vi "Update Calibration.vi"() -> ()   [LabVIEW 2019]
doc: "This VI implements the framework and scheduler for your robotics program. It should not be necessary to modify the framework. You are expected to add your code to the VIs called from Robot Main - the ones located in the Team Code folder within the project."
uses:
  Robot Global Data.vi
panel:
  in  "Color":string(combo)="Red"
  in  "Set Color":bool
  out "Matched Color Name":string
  out "Match Confidence":dbl
  out "Measured Color":cluster{"R":dbl, "G":dbl, "B":dbl}
  in  "Blue Cal":cluster{"R":dbl, "G":dbl, "B":dbl}={"R"=0.143, "G"=0.427, "B"=0.429} caption="Blue Calibration"
  in  "Green Cal":cluster{"R":dbl, "G":dbl, "B":dbl}={"R"=0.197, "G"=0.561, "B"=0.24} caption="Green Calibration"
  in  "Red Cal":cluster{"R":dbl, "G":dbl, "B":dbl}={"R"=0.561, "G"=0.323, "B"=0.114} caption="Red Calibration"
  in  "Yellow Cal":cluster{"R":dbl, "G":dbl, "B":dbl}={"R"=0.361, "G"=0.524, "B"=0.113} caption="Yellow Calibration"
  out "error out":errorcluster
  out "Proximity":u16(graph)
  out "Color":u32(colorbox)
  in  "Finish":bool
  # "To save calibration:\n\nEdit --> Make Current Values Default"
  # "------>"
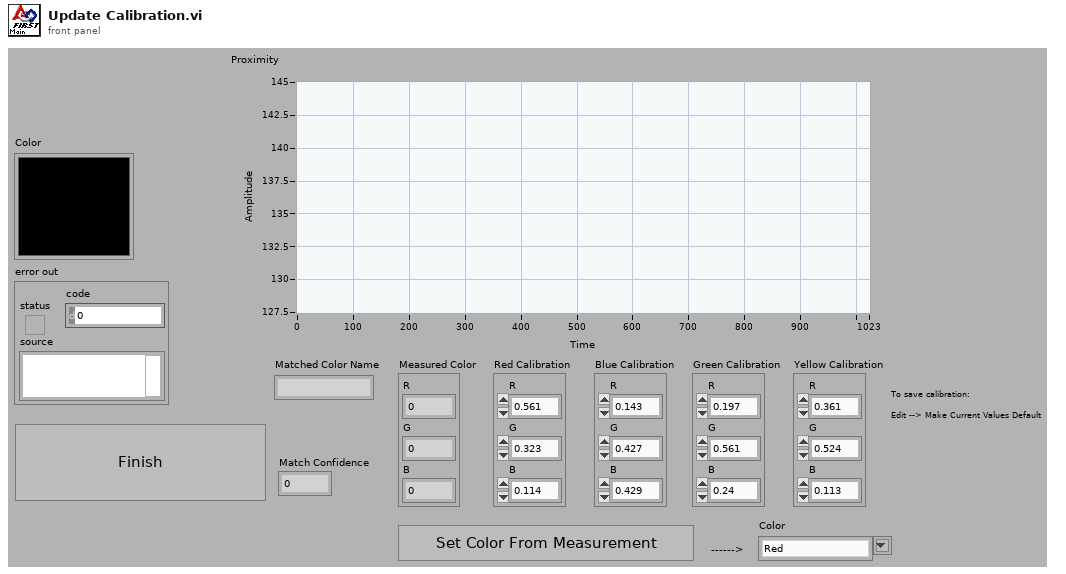
[diagram p1: front panel]
types:
  T1 = typedef "Color Sensor V3 DevRef.ctl" = cluster{"I2CDevRef":T2}
  T2 = typedef "WPI_I2CDevRef.ctl" = cluster{"DevStatus":errorcluster, "Device Address":u8, "Handle":i32, "I2C Bus":T3}
  T3 = typedef "i2c_bus.ctl" = enum16{"I2C On-Board", "I2C MXP", "Invalid"}
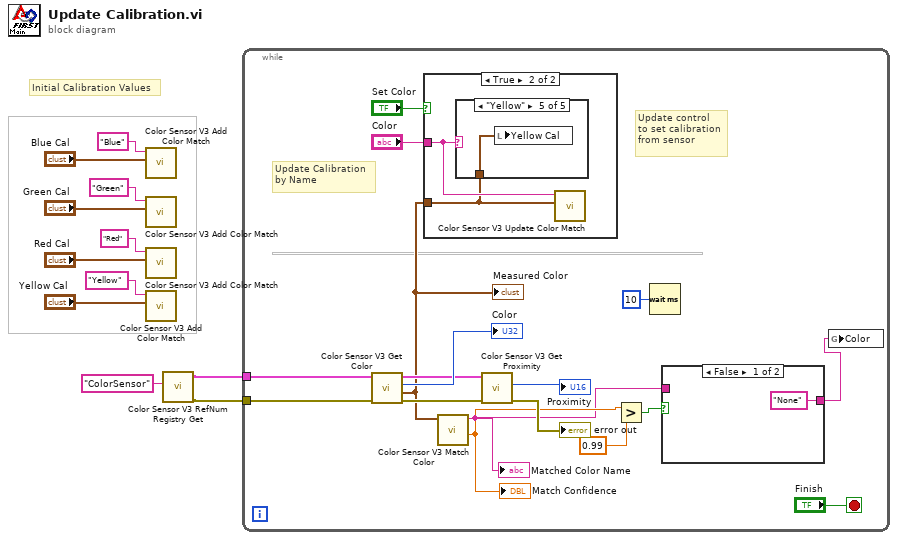
[diagram p0: block diagram]
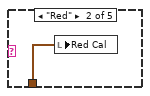
[diagram p5: hidden frame]
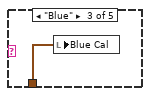
[diagram p6: hidden frame]
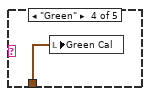
[diagram p7: hidden frame]
diagram:
  # "Initial Calibration Values"
  n1 = call <vilib>:"Color Sensor V3 Add Color Match.vi"("Color"="Blue Cal", "Name"="Blue") -> ()  [unwired: 10 in]
  n2 = call <vilib>:"Color Sensor V3 Add Color Match.vi"("Color"="Green Cal", "Name"="Green") -> ()  [unwired: 10 in]
  n3 = call <vilib>:"Color Sensor V3 Add Color Match.vi"("Color"="Red Cal", "Name"="Red") -> ()  [unwired: 10 in]
  n4 = call <vilib>:"Color Sensor V3 Add Color Match.vi"("Color"="Yellow Cal", "Name"="Yellow") -> ()  [unwired: 10 in]
  n5 = call <vilib>:"Color Sensor V3 RefNum Registry Get.vi"("refnum name"="ColorSensor") -> ("error out"=w2:errorcluster, "ColorSensorDevRef"=w3:T1)  [unwired: 9 in]
  n6 = while "Scheduling loop" {
    tunnel: w3 -> [w18]
    tunnel: w2 -> [w21]
    stop <- "Finish" stop-if-true
    # "Update control\nto set calibration\nfrom sensor"
    # "Update Calibration\nby Name"
    n7 = call <vilib>:"Color Sensor V3 Get Color.vi"("error in (no error)"=w21, "ColorSensorDevRef"=w18) -> ("error out"=w26:errorcluster, "Normalized Color"=w17:cluster{"R":dbl, "G":dbl, "B":dbl}, "Color"=→"Color":u32, "ColorSensorDevRef out"=w25:T1)  [unwired: 6 in]
    "Measured Color" <- w17
    n8 = case shown="True" "Set Color" {
      tunnel: "Color" -> [_ w32]
      tunnel: w17 -> [_ w31]
      frame False {
      }
      frame True {
        n9 = case shown="\"Yellow\"" w32 {
          tunnel: w31 -> [_ w33 w34 w35 w36]
          frame Default {
          }
          frame "Red" {
            n10 = local write "Red Cal"(w33) -> ()
          }
          frame "Blue" {
            n11 = local write "Blue Cal"(w34) -> ()
          }
          frame "Green" {
            n12 = local write "Green Cal"(w35) -> ()
          }
          frame "Yellow" {
            n13 = local write "Yellow Cal"(w36) -> ()
          }
        }
        n14 = call <vilib>:"Color Sensor V3 Update Color Match.vi"("Color"=w31, "Name"=w32) -> ()  [unwired: 10 in]
      }
    }
    n15 = call <vilib>:"Color Sensor V3 Match Color.vi"("Measured Color"=w17) -> ("Confidence"=w16:dbl, "Matched Color Name"=w12:string)  [unwired: 8 in, 1 out]
    "Match Confidence" <- w16
    "Matched Color Name" <- w12
    n16 = call <vilib>:"Color Sensor V3 Get Proximity.vi"("error in (no error)"=w26, "ColorSensorDevRef"=w25) -> ("error out"=→"error out":errorcluster, "Proximity"=→"Proximity":u16)  [unwired: 7 in, 1 out]
    n17 = Greater?(x=w16, y=0.99) -> (0:w15:bool)
    n18 = Wait (ms)(milliseconds to wait=u32 10) -> ()  [unwired: 1 out]
    n19 = case shown="False" w15 {
      tunnel: ["None" ("Matched Color Name") w30] -> w13
      tunnel: w12 -> [_ w30]
      frame False {
      }
      frame True {
      }
    }
    n20 = global write "Robot Global Data.vi" "Color"(w13) -> ()
  }
